vi "DataArrayTest.vi"() -> ()   [LabVIEW 2024]
uses:
  <vilib>/Utility/file.llb/Write Delimited Spreadsheet (string).vi
panel:
  out "appended array 2":string[][](array[string])
  out "output array":string[](array[string])
  out "Array 2":string[](array[string])
  in  "stop":bool
  out "appended array":dbl[][](array[numeric])
  out "Array":dbl[](array[numeric])
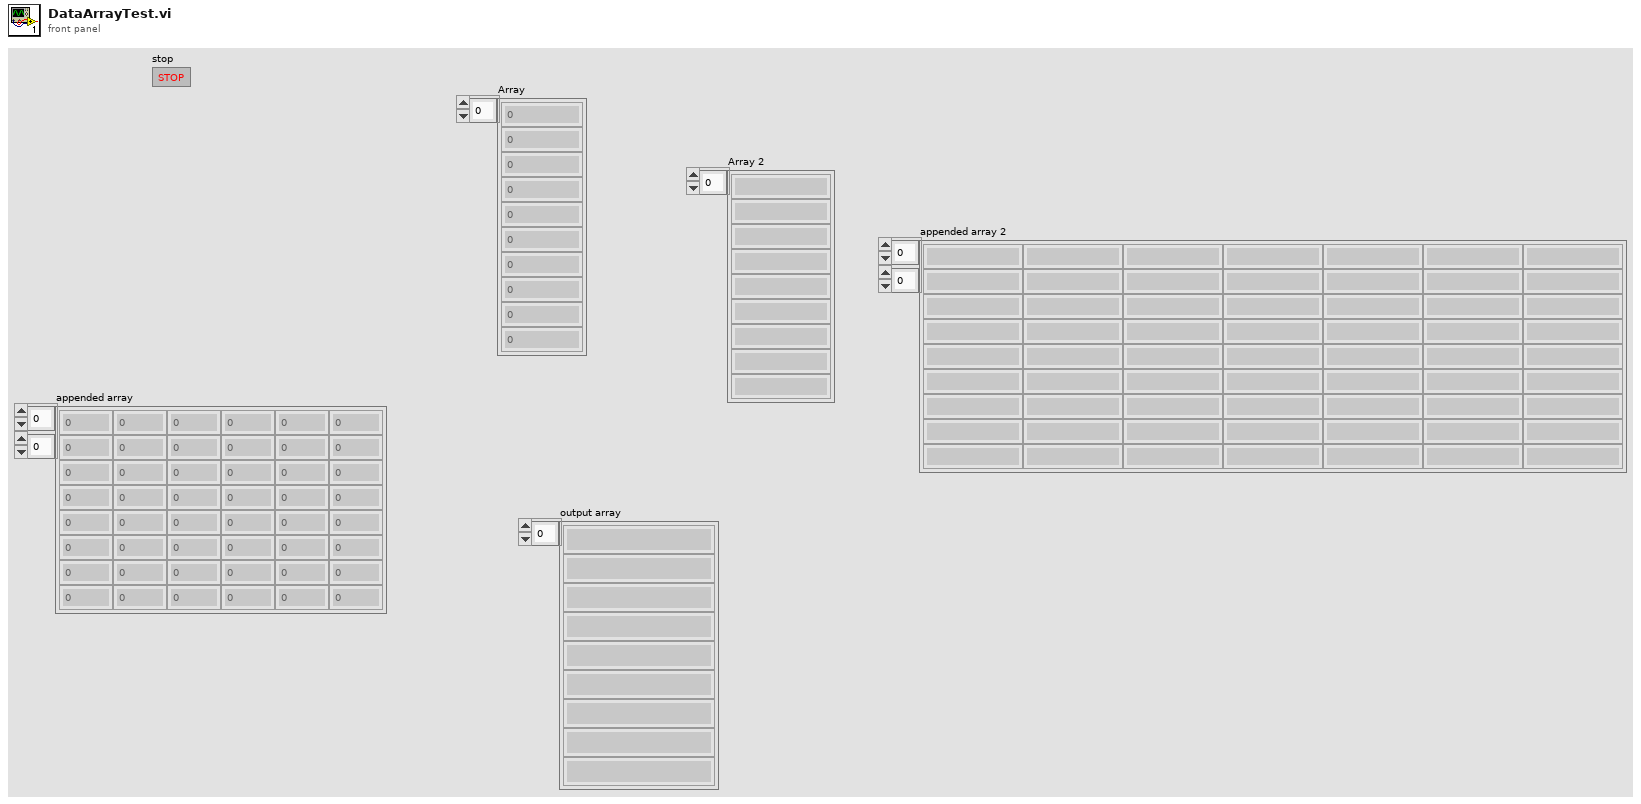
[diagram p1: front panel]
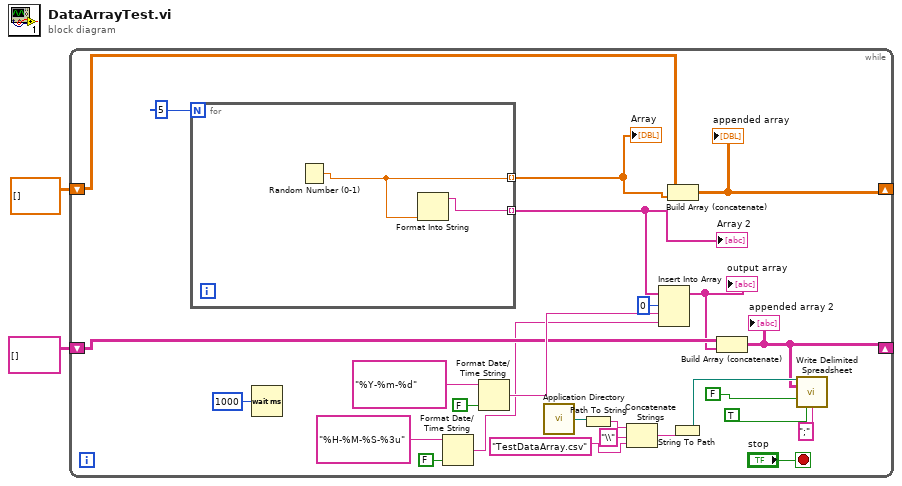
[diagram p0: block diagram]
diagram:
  n1 = while {
    shift-right: [w25] -> _
    shift-left: dbl[][] [] -> [w24]
    shift-right: [w8] -> _
    shift-left: string[][] [] -> [w18]
    stop <- "stop" stop-if-true
    n2 = for {
      N: 5 -> [_]
      tunnel: [w30] -> w26 mode=indexing
      tunnel: [w29] -> w21 mode=indexing
      n3 = Random Number (0-1)() -> (number: 0 to 1=w30:dbl)
      n4 = Format Into String(w30) -> (resulting string=w29:string)  [unwired: 3 in, 1 out]
    }
    "Array" <- w26
    "Array 2" <- w21
    n5 = Wait (ms)(milliseconds to wait=u32 1000) -> ()  [unwired: 1 out]
    n6 = Format Date/Time String(time format string (%c)="%H-%M-%S-%3u", UTC format=FALSE) -> (date/time string=w5:string)  [unwired: 1 in]
    n7 = Format Date/Time String(time format string (%c)="%Y-%m-%d", UTC format=FALSE) -> (date/time string=w19:string)  [unwired: 1 in]
    n8 = call <vilib>:"Application Directory.vi"() -> ("Application Directory"=w16:path)
    n9 = Path To String(path=w16) -> (string=w15:string)
    n10 = Concatenate Strings(w15, "\\" ("string"), "TestDataArray.csv" ("string")) -> (w14:string)
    n11 = Insert Into Array(array=w21, index=0, new element #1=w19, new element #2=w5) -> (w10:string[])
    "output array" <- w10
    n12 = Build Array (concatenate)(w24, w26) -> (w25:dbl[][])
    "appended array" <- w25
    n13 = String To Path(string=w14) -> (path=w13:path)
    n14 = Build Array (concatenate)(w18, w10) -> (w8:string[][])
    "appended array 2" <- w8
    n15 = call-poly <vilib>:"Write Delimited Spreadsheet.vi"("file path (dialog if empty)"=w13, "2D data"=w8, "append to file? (new file:F)"=FALSE, "transpose? (no:F)"=TRUE, "delimiter (\\t)"=";" ("delimiter (\\t)")) -> ()  [unwired: 9 in, 2 out]
  }
